vi "9.vi"() -> ()   [LabVIEW 2017, in "ErrorStructureDrawer-Tests.lvlib"]
uses:
  ErrorStructureDrawer-Tests.lvlib
panel:
  in  "Array":cluster{dbl}[](array[cluster])
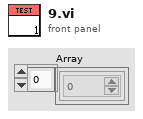
[diagram p1: front panel]
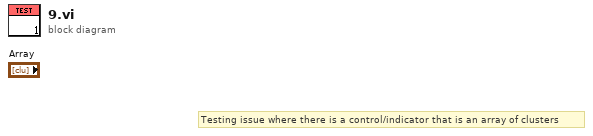
[diagram p0: block diagram]
diagram:
  # "Testing issue where there is a control/indicator that is an array of clusters"
